vi "pp2_stateToDOInt.vi"(11 "State In":T1={"Curr  tr"=0, "Curr (ms)"=0, "Cum (ms)"=0, "Run loop diff"=0, "Tone countdown (ms)"=0, "Countdown (ms)"=0, "Curr State"=enum."0 NULL", "Prev State"=enum."0 NULL", "Null"=FALSE, "Sw1"=FALSE, "Sw2"=FALSE, "Tone\nGate"=FALSE, "Stim"=FALSE, "Current DAQ DO Int"=0, "Current Loaded Trial"={"Trial Type Number"=1, "Trial Type"=enum."GO", "Trial Weight"=100, "Shock (mA)"=0.3, "Duration (ms)"=0.25, "Sound Type"=enum."04 FM Sweep", "Stim P1"=4000.0, "Stim P2"=0.0, "Stim P3"=0.0, "Stim P4"=2000.0}, "Next Trial (for display purposes)"={"Trial Type Number"=1, "Trial Type"=enum."GO", "Trial Weight"=100, "Shock (mA)"=0.3, "Duration (ms)"=0.25, "Sound Type"=enum."04 FM Sweep", "Stim P1"=4000.0, "Stim P2"=0.0, "Stim P3"=0.0, "Stim P4"=2000.0}, "Total trials memo"=0, "State start cum memo (ms)"=0, "Last dur jump time memo (ms)"=0, "Last dur shock time memo (ms)"=0, "Tone repeat memo"=0, "Webcam on"=FALSE, "Webcam recording"=FALSE} {"Current DAQ DO Int" format="%b"; "Next Trial (for display purposes)"."Shock (mA)" min=-1.0 max=5.0; "Next Trial (for display purposes)"."Trial Weight" step=1; "Next Trial (for display purposes)"."Duration (ms)" min=0.0 max=1.0; "Next Trial (for display purposes)"."Trial Type Number" min=1 step=1; "Current Loaded Trial"."Shock (mA)" min=-1.0 max=5.0; "Current Loaded Trial"."Trial Weight" step=1; "Current Loaded Trial"."Duration (ms)" min=0.0 max=1.0; "Current Loaded Trial"."Trial Type Number" min=1 step=1}) -> (3 "DAQ Output Int":u16 format="%b")   [LabVIEW 2013]
uses:
  pp2_CTL_StateInfo.ctl
  pp2_CTL_State.ctl
  pp2_Trial.ctl
  pp2_CTL_TrialType.ctl
  labolabo2/waveforms/WFTypes.ctl
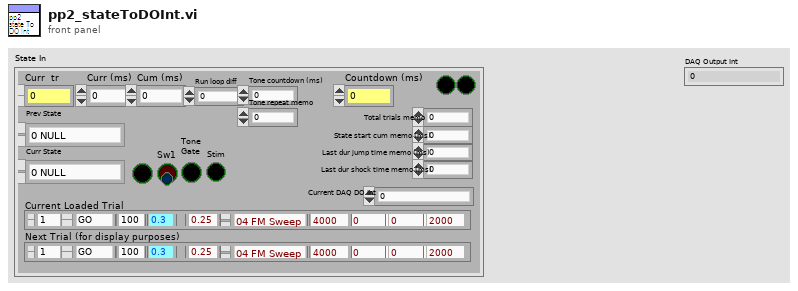
[diagram p1: front panel]
types:
  T1 = typedef "pp2_CTL_StateInfo.ctl" = cluster{"Curr  tr":u16, "Curr (ms)":i64, "Cum (ms)":i64, "Run loop diff":i64, "Tone countdown (ms)":i64, "Countdown (ms)":i64, "Curr State":T2, "Prev State":T2, "Null":bool, "Sw1":bool, "Sw2":bool, "Tone\nGate":bool, "Stim":bool, "Current DAQ DO Int":u16, "Current Loaded Trial":T3, "Next Trial (for display purposes)":T3, "Total trials memo":i64, "State start cum memo (ms)":i64, "Last dur jump time memo (ms)":i64, "Last dur shock time memo (ms)":i64, "Tone repeat memo":i64, "Webcam on":bool, "Webcam recording":bool}
  T2 = typedef "pp2_CTL_State.ctl" = enum8{"0 NULL", "1 Habituation", "2 (Load Trial)", "3 Stay Period", "4 Load Audio/Click Delay", "5 GO Trial", "6 GO Jumped", "7 GO Timeout", "8 NOGO Trial", "9 NOGO Jumped", "10 NOGO Timeout", "11 TEST Trial", "12 TEST Jumped", "13 TEST Timeout", "14 Intertrial Interval", "15 Done"}
  T3 = typedef "pp2_Trial.ctl" = cluster{"Trial Type Number":u8, "Trial Type":T4, "Trial Weight":u32, "Shock (mA)":dbl, "Duration (ms)":dbl, "Sound Type":T5, "Stim P1":dbl, "Stim P2":dbl, "Stim P3":dbl, "Stim P4":dbl}
  T4 = typedef "pp2_CTL_TrialType.ctl" = enum16{"OFF", "GO", "NOGO", "TEST"}
  T5 = typedef "WFTypes.ctl" = enum16{"00 NULL", "01 DC", "02 Noise", "03 Pure Tone", "04 FM Sweep"}
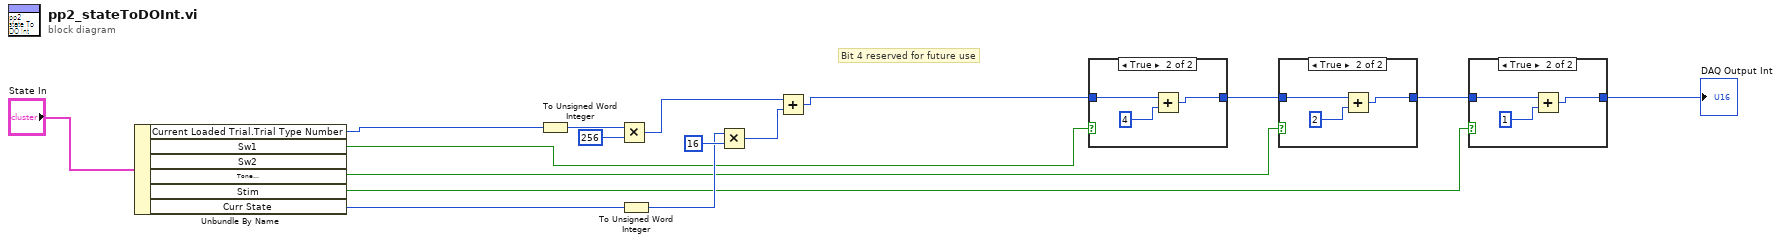
[diagram p0: block diagram]
diagram:
  # "Bit 4 reserved for future use"
  n1 = Unbundle By Name("State In") -> ("Current Loaded Trial.Trial Type Number"=w14:u8, "Sw1"=w3:bool, "Tone\nGate"=w4:bool, "Stim"=w5:bool, "Curr State"=w10:T2)  [unwired: 1 out]
  n2 = To Unsigned Word Integer(number=w14) -> (unsigned 16bit integer=w13:u16)
  n3 = Multiply(x=w13, y=u16 256) -> (x*y=w7:u16)
  n4 = To Unsigned Word Integer(number=w10) -> (unsigned 16bit integer=w8:u16)
  n5 = Multiply(x=w8, y=u16 16) -> (x*y=w6:u16)
  n6 = Add(x=w7, y=w6) -> (x+y=w2:u16)
  n7 = case shown="True" w3 {
    tunnel: [w17 w19] -> w12
    tunnel: w2 -> [w17 w18]
    frame False {
    }
    frame True {
      n8 = Add(x=w18, y=u16 4 ("Current DAQ Digital Out")) -> (x+y=w19:u16)
    }
  }
  n9 = case shown="True" w4 {
    tunnel: w12 -> [w21 w23]
    tunnel: [w21 w22] -> w11
    frame False {
    }
    frame True {
      n10 = Add(x=w23, y=u16 2 ("Current DAQ Digital Out")) -> (x+y=w22:u16)
    }
  }
  n11 = case shown="True" w5 {
    tunnel: w11 -> [w25 w27]
    tunnel: [w25 w26] -> w1
    frame False {
    }
    frame True {
      n12 = Add(x=w27, y=u16 1 ("Current DAQ Digital Out")) -> (x+y=w26:u16)
    }
  }
  "DAQ Output Int" <- w1
